vi "Result_Test.vi"(8 "error in (no error)":errorcluster caption="entrée d'erreur (pas d'erreur)", 11 "Flash_Jlink en entrée":refnum<class "Flash_AVRDUDE.lvclass">) -> (0 "error out":errorcluster caption="sortie d'erreur", 3 "Flash_Jlink en sortie":refnum<class "Flash_AVRDUDE.lvclass">)   [LabVIEW 2020, in "Library Test.lvlib" / "Flash_AVRDUDE.lvclass"]
uses:
  Flash_AVRDUDE.lvclass
  C:/Users/ngarcin/OneDrive - Altyor/Standard TB/Class/Test/Test (Default)/Test (Default).lvclass
  Test_Without_Instr/Test_Without_Inst.lvclass
  Flash_AVRDUDE.lvclass/Flash_AVRDUDE.ctl
panel:
  out "standard output":string caption="sortie standard"
  out "Ok":bool
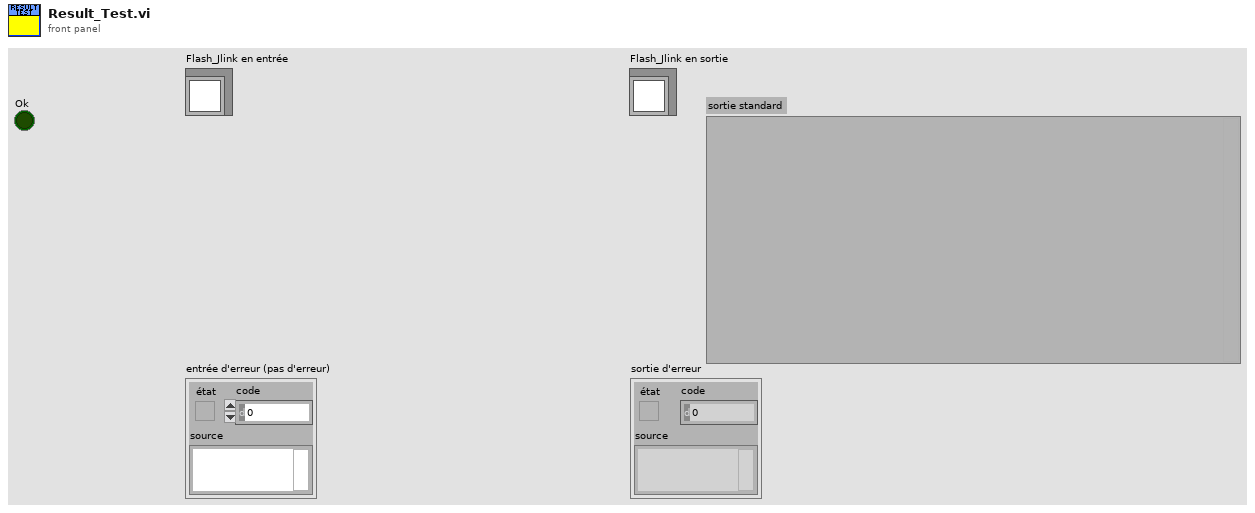
[diagram p1: front panel]
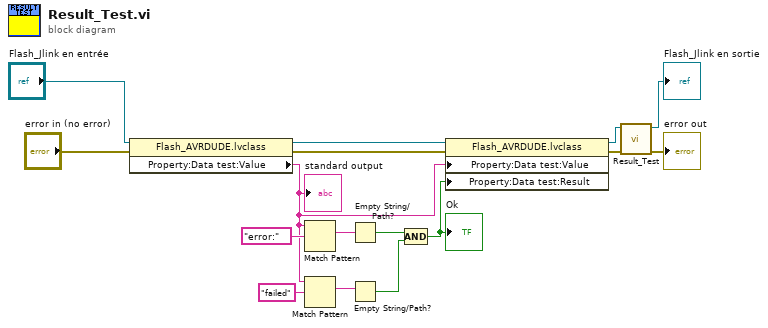
[diagram p0: block diagram]
diagram:
  n1 = property class="Flash_AVRDUDE.lvclass"(reference="Flash_Jlink en entrée", error in="error in (no error)") -> (reference out=w5:refnum<class "Flash_AVRDUDE.lvclass">, error out=w7:errorcluster, "Property:Data test:Value"=w3:string)
  "standard output" <- w3
  n2 = Match Pattern(string=w3, regular expression="error:" ("expression régulière")) -> (match substring=w16:string)  [unwired: 1 in, 3 out]
  n3 = Match Pattern(string=w3, regular expression="failed" ("expression régulière")) -> (match substring=w4:string)  [unwired: 1 in, 3 out]
  n4 = Empty String/Path?(string/path=w16) -> (empty?=w14:bool)
  n5 = Empty String/Path?(string/path=w4) -> (empty?=w1:bool)
  n6 = Compound Arithmetic op=AND(w14, w1) -> (w13:bool)
  "Ok" <- w13
  n7 = property class="Flash_AVRDUDE.lvclass"(reference=w5, error in=w7, "Property:Data test:Value"=w3, "Property:Data test:Result"=w13) -> (reference out=w9:refnum<class "Flash_AVRDUDE.lvclass">, error out=w12:errorcluster)
  n8 = call-parent "Result_Test.vi"("error in (no error)"=w12, "Test_Without_Inst en entrée"=w9) -> ("error out"=→"error out":errorcluster, "Test_Without_Inst en sortie"=→"Flash_Jlink en sortie":refnum<class "Flash_AVRDUDE.lvclass">)  [unwired: 8 in]
